vi "Find Path.vi"(8 "error in (no error)":errorcluster, 9 "channel 2":string, 10 "channel 1":string, 11 "SLSC Switch in":refnum<class "SLSC Switch.lvclass">) -> (0 "error out":errorcluster, 2 "Relay Indexes":i32[](array[numeric]), 3 "SLSC Switch out":refnum<class "SLSC Switch.lvclass">)   [LabVIEW 2016, in "SLSC Switch.lvlib" / "SLSC Switch.lvclass"]
uses:
  SLSC Switch.lvclass
  SLSC Switch.lvclass/SLSC Switch.ctl
  Relay/Relay.lvclass/Relay.ctl
  Relay/Read relay name.vi
  Switch Action Processor/Switch Action Processor.lvclass
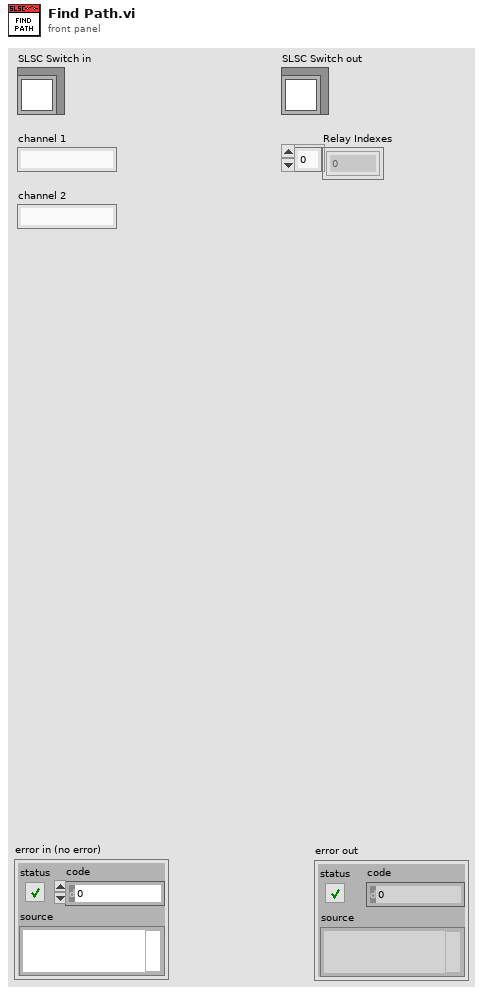
[diagram p1: front panel]
types:
  T1 = typedef "SLSC Switch.lvlib/SLSC Switch.lvclass/Topology.ctl" = cluster{"name":string, "InitialState":T2, "ChannelList":T3, "ConnectionList":T4[], "MuxList":cluster{"Src":string, "Dests":string[]}[]}
  T2 = typedef "SLSC Switch.lvlib/SLSC Switch.lvclass/JSON.InitialState.ctl" = cluster{"Open":string[], "Close":string[]}
  T3 = typedef "SLSC Switch.lvlib/SLSC Switch.lvclass/JSON.ChannelList.ctl" = cluster{"Names":string[]}
  T4 = typedef "SLSC Switch.lvlib/SLSC Switch.lvclass/JSON.ConnectionList.ctl" = cluster{"Src":string, "Dest":string, "Relays":string[]}
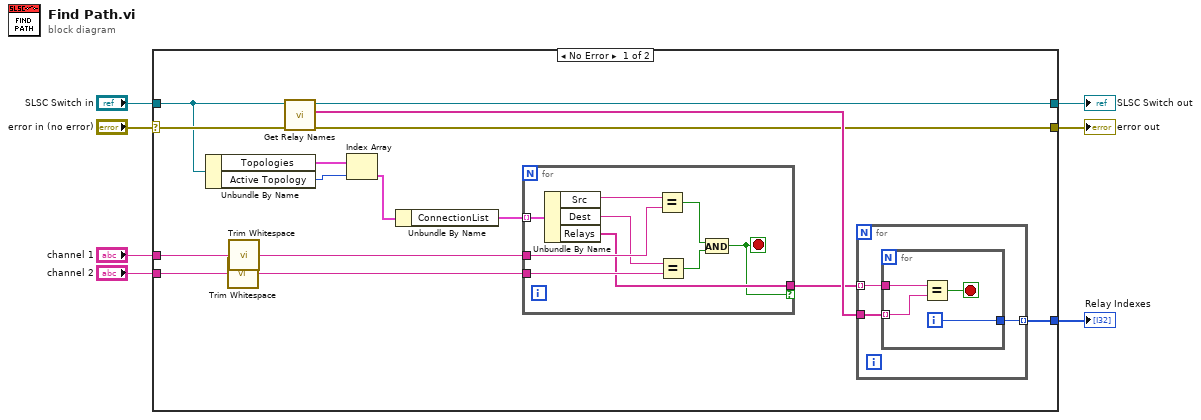
[diagram p0: block diagram]
diagram:
  n1 = case shown="No Error" "error in (no error)" {
    selector: "error in (no error)" -> [w18 w39]
    tunnel: [w22 _] -> w7
    tunnel: [w20 w40] -> w6
    tunnel: "SLSC Switch in" -> [w15 w40]
    tunnel: "channel 2" -> [w9 _]
    tunnel: "channel 1" -> [w11 _]
    tunnel: [w17 w39] -> w1
    frame No Error {
      n2 = Unbundle By Name(w15) -> ("Topologies"=w14:T1[], "Active Topology"=w16:i32)
      n3 = call <vilib>:"Trim Whitespace.vi"("string"=w9) -> ("trimmed string"=w8:string)  [unwired: 1 in]
      n4 = call <vilib>:"Trim Whitespace.vi"("string"=w11) -> ("trimmed string"=w10:string)  [unwired: 1 in]
      n5 = call "Get Relay Names.vi"("error in (no error)"=w18, "SLSC Switch in"=w15) -> ("error out"=w17:errorcluster, "Relay Names"=w21:string[], "SLSC Switch out"=w20:refnum<class "SLSC Switch.lvclass">)  [unwired: 7 in]
      n6 = Index Array(array=w14, index=w16) -> (element=w12:T1)
      n7 = Unbundle By Name(w12) -> ("ConnectionList"=w13:T4[])
      n8 = for {
        tunnel: w13 -> [w31] mode=indexing
        tunnel: w10 -> [w29]
        tunnel: w8 -> [w27]
        tunnel: [w24] -> w19 if=w23
        stop <- w23 stop-if-true
        n9 = Unbundle By Name(w31) -> ("Src"=w30:string, "Dest"=w28:string, "Relays"=w24:string[])
        n10 = Equal?(x=w30, y=w29) -> (x = y?=w26:bool)
        n11 = Equal?(x=w28, y=w27) -> (x = y?=w25:bool)
        n12 = And(x=w26, y=w25) -> (x .and. y?=w23:bool)
      }
      n13 = for {
        tunnel: w19 -> [w33] mode=indexing
        tunnel: w21 -> [w34]
        tunnel: [w32] -> w22 mode=indexing
        n14 = for {
          tunnel: w34 -> [w38] mode=indexing
          tunnel: w33 -> [w37]
          tunnel: [w35] -> w32
          i -> [w35]
          stop <- w36 stop-if-true
          n15 = Equal?(x=w37, y=w38) -> (x = y?=w36:bool)
        }
      }
    }
    frame Error {
    }
  }
  "Relay Indexes" <- w7
  "SLSC Switch out" <- w6
  "error out" <- w1
